vi "Pre-Process.vi"(11 "Main Controller Actor in":refnum<class "Main Controller Actor.lvclass">) -> (3 "Main Controller Actor out":refnum<class "Main Controller Actor.lvclass">)   [LabVIEW 2021, in "Main Controller Actor.lvclass"]
uses:
  Main Controller Actor.lvclass
  Main Controller Actor.lvclass/Main Controller Actor.ctl
  Element/Element.lvclass
  Globals.vi
  1a8e91d4-f7ca-4908-87bb-deb0e57cb28f.vi
  3f9179ff-e07b-42f4-a04d-d75a8adb2856.vi
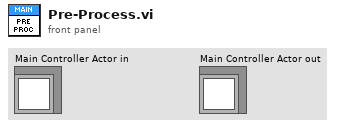
[diagram p1: front panel]
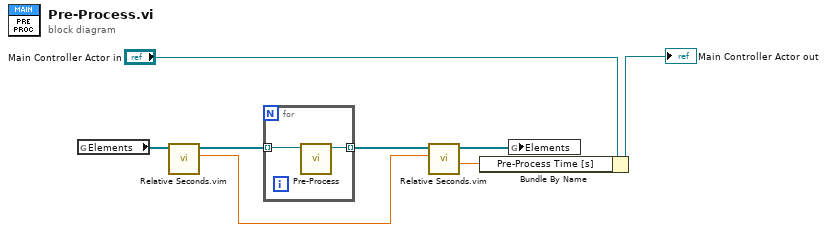
[diagram p0: block diagram]
diagram:
  n1 = global read "Globals.vi" "Elements"() -> (w6:refnum<class "Element.lvclass">[])
  n2 = call "Relative Seconds.vim"("Anything in"=w6) -> ("Relative Seconds out"=w2:dbl, "Anything out"=w5:refnum<class "Element.lvclass">[])  [unwired: 8 in, 1 out]
  n3 = for {
    tunnel: [w10] -> w4 mode=indexing
    tunnel: w5 -> [w9] mode=indexing
    n4 = call-dynamic "Pre-Process.vi"("Element in"=w9) -> ("Element out"=w10:refnum<class "Element.lvclass">)  [unwired: 10 in]
  }
  n5 = call "Relative Seconds.vim"("Relative Seconds in"=w2, "Anything in"=w4) -> ("Relative Seconds delta"=w1:dbl, "Anything out"=w3:refnum<class "Element.lvclass">[])  [unwired: 7 in, 1 out]
  n6 = Bundle By Name(cluster="Main Controller Actor in", "Pre-Process Time [s]"=w1) -> (→"Main Controller Actor out":refnum<class "Main Controller Actor.lvclass">)
  n7 = global write "Globals.vi" "Elements"(w3) -> ()
